vi "PwF_ToF_ConfigRanging.vi"(0 "PwF ToF Ref":T1, 5 "Ranging Mode":T2, 7 "Tsamp_ms":u16=50, 9 "ROI_TL_Xcoord":u8=255, 11 "error in (no error)":errorcluster, 12 "ROI_TL_Ycoord":u8=255, 13 "ROI_BR_Xcoord":u8=255, 14 "ROI_BR_Ycoord":u8=255) -> (4 "PwF ToF Ref":T1, 15 "error out":errorcluster)   [LabVIEW 2018]
uses:
  ToF_TypeDef/PwF ToF Ref.ctl
  ToF_TypeDef/PwF ToF RangingMode.ctl
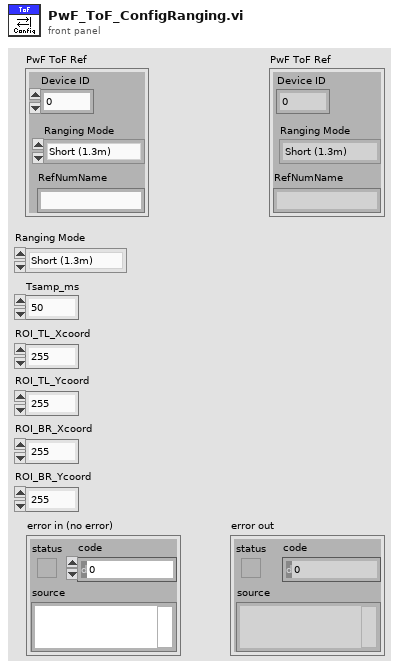
[diagram p1: front panel]
types:
  T1 = typedef "PwF ToF Ref.ctl" = cluster{"Device ID":u8, "Ranging Mode":T2, "RefNumName":string}
  T2 = typedef "PwF ToF RangingMode.ctl" = enum8{"Short (1.3m)", "Medium (2m)", "Long (4m)"}
  T3 = cluster{u8, u8, u8, "ROI_TL_Xcoord":u8, "ROI_TL_Ycoord":u8, "ROI_BR_Xcoord":u8, "ROI_BR_Ycoord":u8}
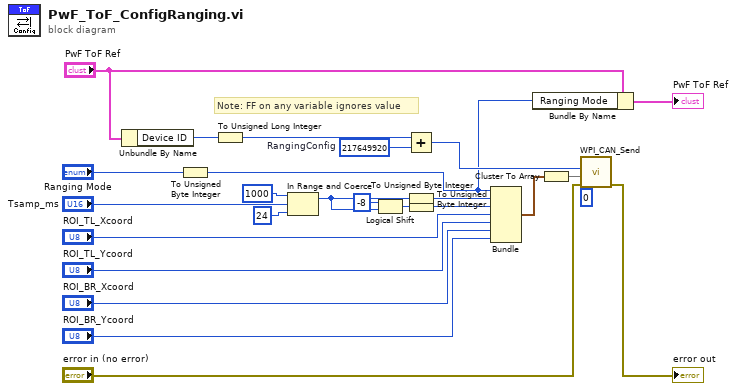
[diagram p0: block diagram]
diagram:
  w25 = u32 217649920  # RangingConfig
  # "Note: FF on any variable ignores value"
  n1 = Unbundle By Name("PwF ToF Ref") -> ("Device ID"=w2:u8)
  n2 = To Unsigned Byte Integer(number="Ranging Mode") -> (unsigned 8bit integer=w4:u8)
  n3 = To Unsigned Long Integer(number=w2) -> (unsigned 32bit integer=w1:u32)
  n4 = In Range and Coerce(upper limit=u16 1000, x="Tsamp_ms", lower limit=u16 24) -> (coerced(x)=w16:u16)  [unwired: 1 out]
  n5 = Logical Shift(y=i16 -8, x=w16) -> (x << y=w23:u16)
  n6 = Add(x=w1, y=w25) -> (x+y=w17:u32)
  n7 = To Unsigned Byte Integer(number=w16) -> (unsigned 8bit integer=w22:u8)
  n8 = To Unsigned Byte Integer(number=w23) -> (unsigned 8bit integer=w21:u8)
  n9 = Bundle(w4, w22, w21, "ROI_TL_Xcoord"="ROI_TL_Xcoord", "ROI_TL_Ycoord"="ROI_TL_Ycoord", "ROI_BR_Xcoord"="ROI_BR_Xcoord", "ROI_BR_Ycoord"="ROI_BR_Ycoord") -> (w19:T3)  [unwired: 1 in]
  n10 = Bundle By Name(cluster="PwF ToF Ref", "Ranging Mode"=w4) -> (→"PwF ToF Ref":T1)
  n11 = Cluster To Array(cluster=w19) -> (array=w20:u8[])
  n12 = call <vilib>:"WPI_CAN_Send.vi"("Period (ms)"=0, "error in (no error)"="error in (no error)", "Data"=w20, "Message ID"=w17) -> ("error out"=→"error out":errorcluster)  [unwired: 7 in]
